vi "CopyAttributes.vi"(8 "error in (no error)":errorcluster, 10 "Attributes":variant, 11 "BrowerComposite in":refnum<class "BrowerComposite.lvclass">) -> (0 "error out":errorcluster, 3 "BrowerComposite out":refnum<class "BrowerComposite.lvclass">)   [LabVIEW 2015, in "BrowerComposite.lvclass"]
uses:
  BrowerComposite.lvclass
  BrowerComposite.lvclass/BrowerComposite.ctl
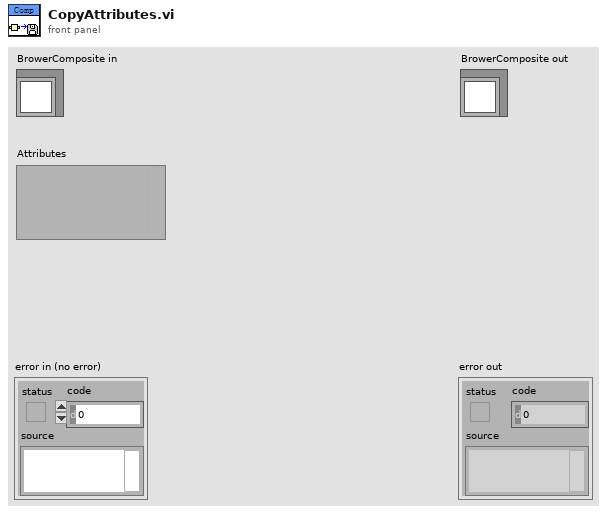
[diagram p1: front panel]
types:
  T1 = typedef "BrowerComposite.lvclass/ObjectAttributes.ctl" = cluster{"BrowerComponents":refnum<class "BrowerComponent.lvclass">[], "BrowerComponentIDs":string[], "Iterator":refnum<class "Iterator.lvclass">}
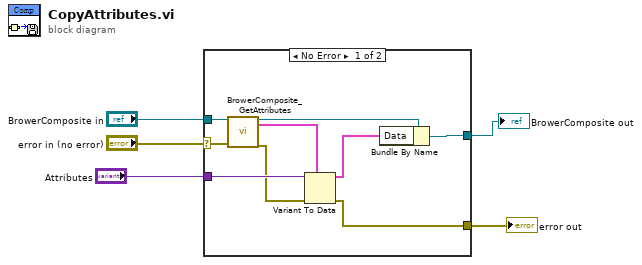
[diagram p0: block diagram]
diagram:
  n1 = case shown="No Error" "error in (no error)" {
    selector: "error in (no error)" -> [w13 w15]
    tunnel: "BrowerComposite in" -> [w14 w16]
    tunnel: [w11 w16] -> w3
    tunnel: [w6 w15] -> w2
    tunnel: "Attributes" -> [w10 _]
    frame No Error {
      n2 = call "BrowerComposite_GetAttributes.vi"("reference in"=w14, "error in (no error)"=w13) -> ("reference out"=w12:refnum<class "BrowerComposite.lvclass">, "Data"=w9:T1, "error out"=w7:errorcluster)  [unwired: 14 in, 1 out]
      n3 = Variant To Data(error in=w7, type=w9, Variant=w10) -> (data=w8:T1, error out=w6:errorcluster)
      n4 = Bundle By Name(cluster=w12, "Data"=w8) -> (w11:refnum<class "BrowerComposite.lvclass">)
    }
    frame Error {
    }
  }
  "error out" <- w2
  "BrowerComposite out" <- w3
